vi "Create CONNECT Packet.vi"(5 "type":refnum<class "CONNECT.lvclass">, 6 "Keep Alive (s)":u16, 7 "Client ID (empty: generate new)":string, 8 "error in (no error)":errorcluster, 10 "Payload":T1, 11 "Connect Flags":T2) -> (0 "error out":errorcluster, 3 "CONNECT":refnum<class "CONNECT.lvclass">)   [LabVIEW 2013, in "CONNECT.lvclass"]
uses:
  CONNECT.lvclass
  ConnectFlags -- cluster.ctl
  CONNECT.lvclass/CONNECT.ctl
  ControlPacket/ControlPacket.lvclass/ControlPacket.ctl
  ControlPacket/ControlPacket.lvclass
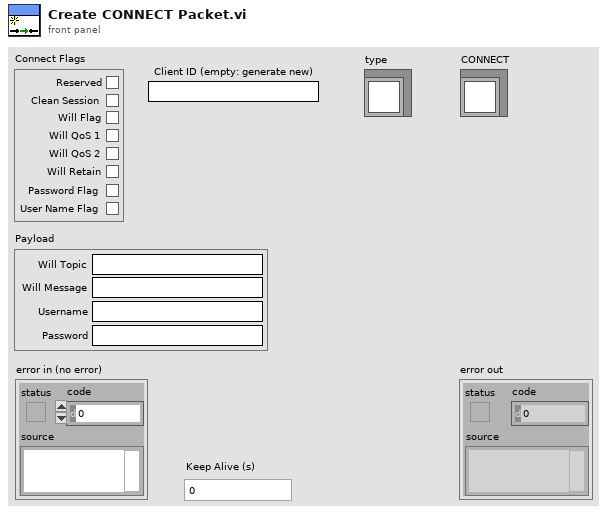
[diagram p1: front panel]
types:
  T1 = cluster{"Will Topic":string, "Will Message":string, "Username":string, "Password":string}
  T2 = typedef "CONNECT.lvclass/ConnectFlags -- cluster.ctl" = cluster{"Reserved":bool, "Clean Session":bool, "Will Flag":bool, "Will QoS 1":bool, "Will QoS 2":bool, "Will Retain":bool, "Password Flag":bool, "User Name Flag":bool}
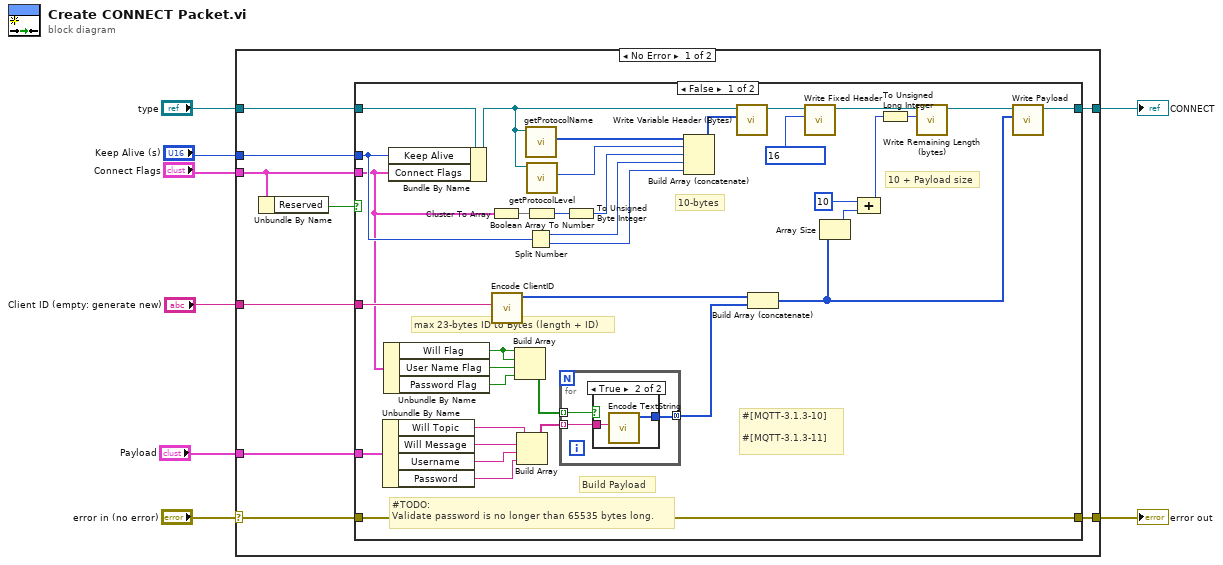
[diagram p0: block diagram]
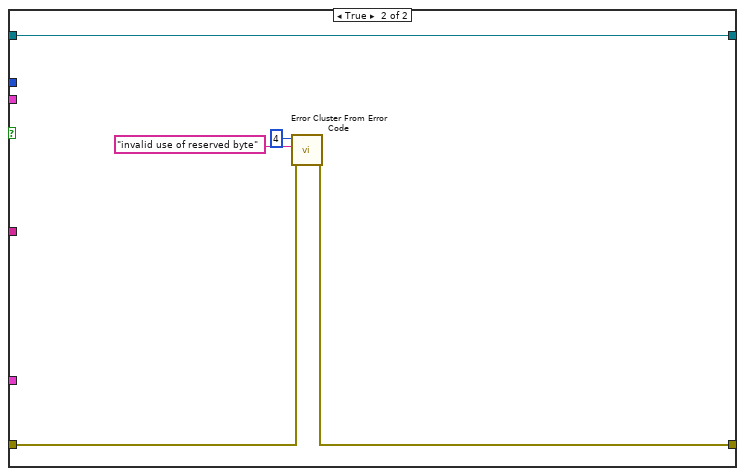
[diagram p3: hidden frame]
diagram:
  n1 = case shown="No Error" "error in (no error)" {
    selector: "error in (no error)" -> [w15 w65]
    tunnel: [w16 w65] -> w7
    tunnel: [w13 w64] -> w5
    tunnel: "type" -> [w14 w64]
    tunnel: "Connect Flags" -> [w12 _]
    tunnel: "Keep Alive (s)" -> [w11 _]
    tunnel: "Client ID (empty: generate new)" -> [w10 _]
    tunnel: "Payload" -> [w9 _]
    frame No Error {
      n2 = Unbundle By Name(w12) -> ("Reserved"=w17:bool)
      n3 = case shown="False" w17 {
        tunnel: [w53 w61] -> w16
        tunnel: w15 -> [w53 w60]
        tunnel: w14 -> [w52 w59]
        tunnel: [w39 w59] -> w13
        tunnel: w12 -> [w32 _]
        tunnel: w11 -> [w45 _]
        tunnel: w10 -> [w34 _]
        tunnel: w9 -> [w33 _]
        frame False {
          # "#TODO: \nValidate password is no longer than 65535 bytes long."
          # "#[MQTT-3.1.3-10]\n\n#[MQTT-3.1.3-11]"
          # "Build Payload"
          # "10-bytes"
          # "max 23-bytes ID to Bytes (length + ID)"
          # "10 + Payload size"
          n4 = Unbundle By Name(w33) -> ("Will Topic"=w28:string, "Will Message"=w27:string, "Username"=w26:string, "Password"=w25:string)
          n5 = Unbundle By Name(w32) -> ("Will Flag"=w31:bool, "User Name Flag"=w30:bool, "Password Flag"=w29:bool)
          n6 = Bundle By Name(cluster=w52, "Keep Alive"=w45, "Connect Flags"=w32) -> (w44:refnum<class "CONNECT.lvclass">)
          n7 = Cluster To Array(cluster=w32) -> (array=w51:bool[])
          n8 = call "Encode ClientID.vi"("Client ID (empty: generate new)"=w34) -> ("Length-Prefixed Field"=w21:u8[])  [unwired: 9 in, 1 out]
          n9 = Build Array(w31, w31, w30, w29) -> (w24:bool[])
          n10 = Build Array(w28, w27, w26, w25) -> (w23:string[])
          n11 = call "getProtocolName.vi"("CONNECT in"=w44) -> ("ProtocolName"=w50:u8[])  [unwired: 9 in, 1 out]
          n12 = Split Number(x=w45) -> (hi(x)=w20:u8, lo(x)=w19:u8)
          n13 = call "getProtocolLevel.vi"("CONNECT in"=w44) -> ("Protocol Level"=w49:u8)  [unwired: 9 in, 1 out]
          n14 = Boolean Array To Number(Boolean array=w51) -> (number=w48:u32)
          n15 = for {
            tunnel: w24 -> [w56] mode=indexing
            tunnel: w23 -> [w55] mode=indexing
            tunnel: [w54] -> w22 mode=concatenating
            n16 = case shown="True" w56 {
              tunnel: w55 -> [_ w58]
              tunnel: [_ w57] -> w54
              frame False {
              }
              frame True {
                n17 = call "Encode TextString.vi"("Text String"=w58) -> ("Length-Prefixed Field"=w57:u8[])  [unwired: 10 in]
              }
            }
          }
          n18 = To Unsigned Byte Integer(number=w48) -> (unsigned 8bit integer=w47:u8)
          n19 = Build Array (concatenate)(w50, w49, w47, w20, w19) -> (w46:u8[])
          n20 = call "Write Variable Header (Bytes).vi"("Variable Header (Bytes)"=w46, "ControlPacket in"=w44) -> ("ControlPacket out"=w43:refnum<class "CONNECT.lvclass">)  [unwired: 9 in]
          n21 = Build Array (concatenate)(w21, w22) -> (w18:u8[])
          n22 = call "Write Fixed Header.vi"("Fixed Header"=u8 16, "ControlPacket in"=w43) -> ("ControlPacket out"=w41:refnum<class "CONNECT.lvclass">)  [unwired: 9 in]
          n23 = Array Size(array=w18) -> (size(s)=w38:i32)
          n24 = Compound Arithmetic op=ADD(10 ("value"), w38) -> (w36:i32)
          n25 = To Unsigned Long Integer(number=w36) -> (unsigned 32bit integer=w35:u32)
          n26 = call "Write Remaining Length (bytes).vi"("Remaining Length (bytes)"=w35, "ControlPacket in"=w41) -> ("ControlPacket out"=w40:refnum<class "CONNECT.lvclass">)  [unwired: 9 in]
          n27 = call "Write Payload.vi"("Payload"=w18, "ControlPacket in"=w40) -> ("ControlPacket out"=w39:refnum<class "CONNECT.lvclass">)  [unwired: 9 in]
        }
        frame True {
          n28 = call <vilib>:"Error Cluster From Error Code.vi"("error in (no error)"=w60, "error message (\"\")"="invalid use of reserved byte" ("error message (\"\")"), "error code (0)"=4) -> ("error out"=w61:errorcluster)  [unwired: 6 in]
        }
      }
    }
    frame Error {
    }
  }
  "error out" <- w7
  "CONNECT" <- w5
